vi "Parse Message.vi"(1 "Controller Message":T2={"MDS Command"=enum."Set VMode", "Channel"=0, "Value"=variant}) -> (5 "MDS Command":T1=enum."Open", 7 "Channel":u8, 8 "Value":variant)   [LabVIEW 2019, in "Controller.lvlib"]
uses:
  Controller.lvlib
  Controller Message.ctl
  MDS Command.ctl
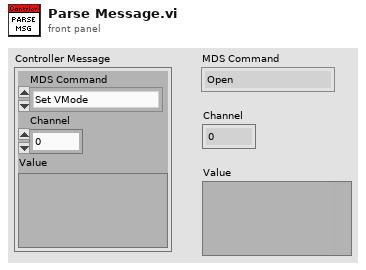
[diagram p1: front panel]
types:
  T1 = typedef "Controller.lvlib/MDS Command.ctl" = enum16{"Idle", "Open", "Set VMode", "Set IMode", "Get Frequency", "Set Frequency", "Get Power", "Set Power (dBm)", "Set Power (%)", "Get Switch", "Switch Channel", "Store", "Wait for Prompt", "Wait for State", "Reset", "Error", "Close", "Stop"}
  T2 = typedef "Controller.lvlib/Controller Message.ctl" = cluster{"MDS Command":T1, "Channel":u8, "Value":variant}
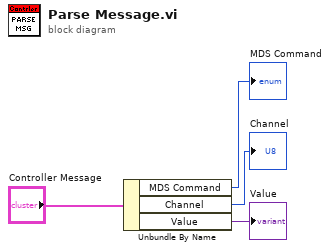
[diagram p0: block diagram]
diagram:
  n1 = Unbundle By Name("Controller Message") -> ("MDS Command"=→"MDS Command":T1, "Channel"=→"Channel":u8, "Value"=→"Value":variant)
